vi "Read Component Operations Errors.vi"(8 "Error In":errorcluster, 11 "Component in":refnum<class "Component.lvclass">) -> (0 "Error Out":errorcluster, 2 "Component Operations Errors":errorcluster, 3 "Component out":refnum<class "Component.lvclass">)   [LabVIEW 2017, in "CL_G3_VIComponentBuilder.lvlib" / "Component.lvclass"]
uses:
  Component.lvclass
  Component.lvclass/Component.ctl
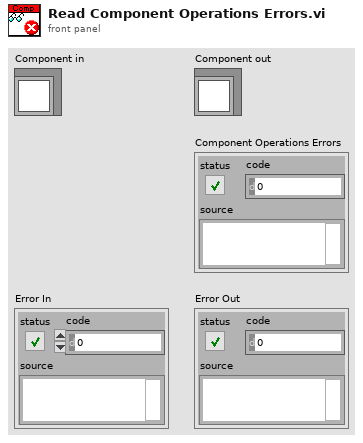
[diagram p1: front panel]
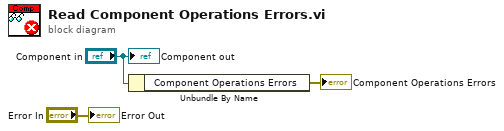
[diagram p0: block diagram]
diagram:
  n1 = Unbundle By Name("Component in") -> ("Component Operations Errors"=→"Component Operations Errors":errorcluster)
  "Component out" <- "Component in"
  "Error Out" <- "Error In"
